vi "Remove a Dev Requested by UI.vi"(8 "error in (no error)":errorcluster, 10 "DevInfo":refnum<class "DevInfo.lvclass">, 11 "Controller in":refnum<class "Controller.lvclass">) -> (0 "error out":errorcluster, 3 "Controller out":refnum<class "Controller.lvclass">)   [LabVIEW 2016, in "Controller Actor.lvlib" / "Controller.lvclass"]
uses:
  <userlib>/Common Components/Controller/Controller.lvclass
  <userlib>/Common Components/Hardware/DevInfo/DevInfo.lvclass
  <userlib>/Common Components/Hardware/DevInfo/DevInfo.lvclass/DevInfo.ctl
  <userlib>/Common Components/Hardware/DevInfo/Read GUID.vi
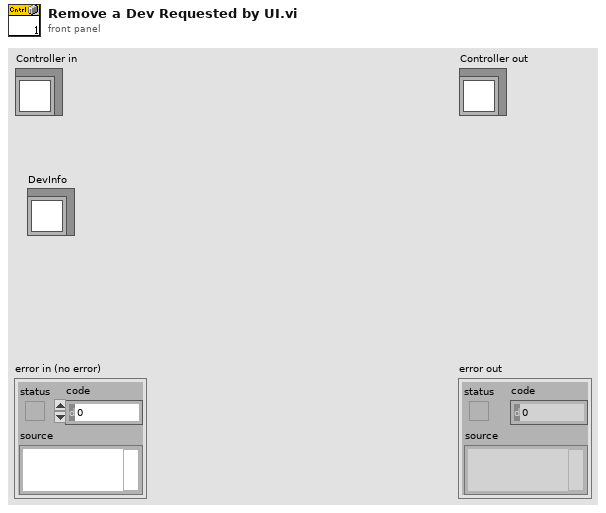
[diagram p1: front panel]
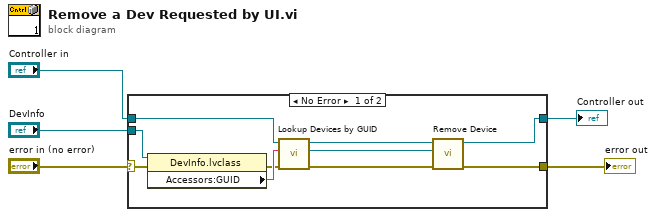
[diagram p0: block diagram]
diagram:
  n1 = case shown="No Error" "error in (no error)" {
    selector: "error in (no error)" -> [w11 w17]
    tunnel: [w9 w17] -> w4
    tunnel: [w7 w16] -> w2
    tunnel: "Controller in" -> [w14 w16]
    tunnel: "DevInfo" -> [w15 _]
    frame No Error {
      n2 = property class="DevInfo.lvclass"(reference=w15, error in=w11) -> (error out=w10:errorcluster, "Accessors:GUID"=w13:string)  [unwired: 1 out]
      n3 = call <userlib>:"Lookup Devices by GUID.vi"("error in (no error)"=w10, "GUID"=w13, "Controller in"=w14) -> ("error out"=w12:errorcluster, "Dev Obj out"=w6:refnum<class "Hardware.lvclass">, "Controller out"=w8:refnum<class "Controller.lvclass">)  [unwired: 6 in]
      n4 = call <userlib>:"Remove Device.vi"("error in (no error)"=w12, "Device"=w6, "Controller in"=w8) -> ("error out"=w9:errorcluster, "Controller out"=w7:refnum<class "Controller.lvclass">)  [unwired: 7 in]
    }
    frame Error {
    }
  }
  "error out" <- w4
  "Controller out" <- w2
